vi "Swerve Wheel 6181.vi"(2 "Wheel":T1(ring), 4 "Inputs":dbl[](array[numeric])) -> (0 "Speed":dbl)   [LabVIEW 2019]
doc: "This vi is used to calculate and control the position of the swerve wheels and the commanded output to the drive motors."
uses:
  <vilib>/Rock Robotics/WPI/Utilities/WPI_GetSetVariantRefNum.vi
  <vilib>/addons/control/pid/pid.llb/PID (DBL).vi
  <vilib>/addons/control/pid/NI_PID_pid.lvlib
panel:
  in  "BR":dbl=245.0 format="%#_13g"
  in  "BL":dbl=95.0 format="%#_13g"
  in  "FR":dbl=267.0 format="%#_13g"
  in  "FL":dbl=75.0 format="%#_13g"
  # "Steering Motor Encoder Offsets"
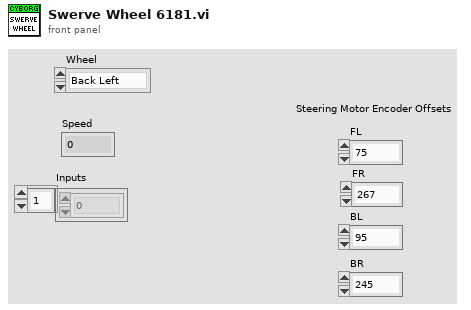
[diagram p1: front panel]
types:
  T1 = enum16{"Back Left", "Back Right", "Front Left", "Front Right"}
  T2 = enum16{"Z", "Y", "X", "Width/2", "Length/2", "Max"}
  T3 = cluster{"proportional gain (Kc)":dbl, "integral time (Ti, min)":dbl, "derivative time (Td, min)":dbl}
  T4 = typedef "WPI_AnalogChannelDevRef.ctl" = cluster{"DevStatus":errorcluster, "Analog Channel":T5}
  T5 = typedef "FPGA_AIChannel.ctl" = enum8{"AI 0", "AI 1", "AI 2", "AI 3", "AI MXP 0", "AI MXP 1", "AI MXP 2", "AI MXP 3", "Invalid"}
  T6 = typedef "WPI_MotorControlDeviceRef.ctl" = cluster{"DeviceStatus":errorcluster, "Type":T7, "PWM":cluster{"PWM Channel":T8, "DeadBand":T9}, "CAN":cluster{"Device Number":u8, "SetOutput VI Ref":variant, "GetOutput VI Ref":variant, "Enable VI Ref":variant, "Disable VI Ref":variant, "Data":variant}, "Invert":bool, "DIO PWM":cluster{"PWM \"Enable\" Channel":T8, "DIOChannel":T10, "PWM Rate":dbl}}
  T7 = typedef "WPI_MotorControlType.ctl" = enum16{"PWM", "CAN", "DIO PWM"}
  T8 = typedef "FPGA_DIOPWMChannel.ctl" = enum8{"PWM 0", "PWM 1", "PWM 2", "PWM 3", "PWM 4", "PWM 5", "PWM 6", "PWM 7", "PWM 8", "PWM 9", "PWM MXP 0", "PWM MXP 1", "PWM MXP 2", "PWM MXP 3", "PWM MXP 4", "PWM MXP 5", "PWM MXP 6", "PWM MXP 7", "PWM MXP 8", "PWM MXP 9", "Invalid"}
  T9 = typedef "WPI_PWMDeadband.ctl" = cluster{"Name":string, "maxPositivePwm":i32, "minPositivePwm":i32, "centerPwm":i32, "maxNegativePwm":i32, "minNegativePwm":i32, "angularRange":u16}
  T10 = typedef "FPGA_DIOChannel.ctl" = enum8{"DIO 0", "DIO 1", "DIO 2", "DIO 3", "DIO 4", "DIO 5", "DIO 6", "DIO 7", "DIO 8", "DIO 9", "DIO MXP 0", "DIO MXP 1", "DIO MXP 2", "DIO MXP 3", "DIO MXP 4", "DIO MXP 5", "DIO MXP 6", "DIO MXP 7", "DIO MXP 8", "DIO MXP 9", "DIO MXP 10", "DIO MXP 11", "DIO MXP 12", "DIO MXP 13", "DIO MXP 14", "DIO MXP 15", "SPI Port CS1", "SPI Port CS2", "SPI Port CS3", "SPI Port MISO", "SPI Port MOSI", "Invalid"}
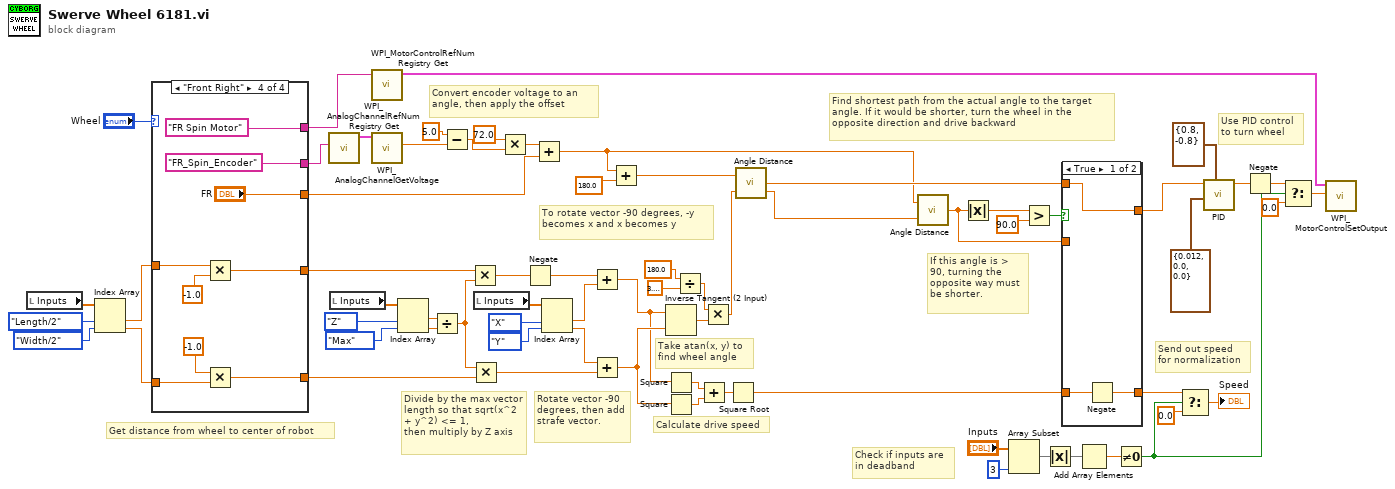
[diagram p0: block diagram]
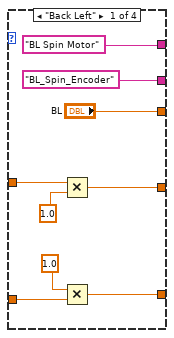
[diagram p3: hidden frame]
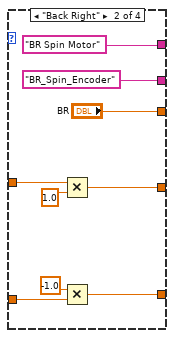
[diagram p4: hidden frame]
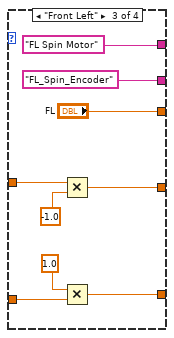
[diagram p5: hidden frame]
diagram:
  # "To rotate vector -90 degrees, -y becomes x and x becomes y"
  # "Divide by the max vector length so that sqrt(x^2 + y^2) <= 1,\nthen multiply by Z axis"
  # "Send out speed\nfor normalization"
  # "Check if inputs are\nin deadband"
  # "Convert encoder voltage to an angle, then apply the offset"
  # "If this angle is > 90, turning the opposite way must be shorter."
  # "Use PID control\nto turn wheel"
  # "Find shortest path from the actual angle to the target angle. If it would be shorter, turn the wheel in the opposite direction and drive backward"
  # "Take atan(x, y) to find wheel angle"
  # "Calculate drive speed"
  # "Rotate vector -90 degrees, then add strafe vector."
  # "Get distance from wheel to center of robot"
  n1 = local read "Inputs"() -> (w20:dbl[])
  n2 = Index Array(array=w20, index #1=T2."Length/2", index #2=T2."Width/2") -> (element #1=w19:dbl, element #2=w18:dbl)
  n3 = case shown="\"Front Right\"" "Wheel" {
    tunnel: ["BL_Spin_Encoder" "BR_Spin_Encoder" "FL_Spin_Encoder" "FR_Spin_Encoder"] -> w4
    tunnel: ["BL Spin Motor" "BR Spin Motor" "FL Spin Motor" "FR Spin Motor"] -> w3
    tunnel: ["BL" "BR" "FL" "FR"] -> w47
    tunnel: w19 -> [w73 w82 w91 w100]
    tunnel: w18 -> [w71 w80 w89 w98]
    tunnel: [w70 w79 w88 w97] -> w34
    tunnel: [w69 w78 w87 w96] -> w33
    frame "Back Left" {
      n4 = Multiply(x=w73, y=1.0) -> (x*y=w70:dbl)
      n5 = Multiply(x=1.0 ("y"), y=w71) -> (x*y=w69:dbl)
    }
    frame "Back Right" {
      n6 = Multiply(x=w82, y=1.0) -> (x*y=w79:dbl)
      n7 = Multiply(x=-1.0 ("y"), y=w80) -> (x*y=w78:dbl)
    }
    frame "Front Left" {
      n8 = Multiply(x=w91, y=-1.0) -> (x*y=w88:dbl)
      n9 = Multiply(x=1.0 ("y"), y=w89) -> (x*y=w87:dbl)
    }
    frame "Front Right" {
      n10 = Multiply(x=w100, y=-1.0) -> (x*y=w97:dbl)
      n11 = Multiply(x=-1.0 ("y"), y=w98) -> (x*y=w96:dbl)
    }
  }
  n12 = call <vilib>:"WPI_AnalogChannelRefNum Registry Get.vi"("refnum name"=w4) -> ("AIDeviceRef"=w50:T4)  [unwired: 9 in, 1 out]
  n13 = local read "Inputs"() -> (w32:dbl[])
  n14 = call <vilib>:"WPI_MotorControlRefNum Registry Get.vi"("refnum name"=w3) -> ("MotorControlDevRef"=w65:T6)  [unwired: 9 in, 1 out]
  n15 = call <vilib>:"WPI_AnalogChannelGetVoltage.vi"("AIDeviceRef"=w50) -> ("Voltage"=w13:dbl)  [unwired: 8 in, 2 out]
  n16 = Index Array(array=w32, index #1=T2."Z", index #2=T2."Max") -> (element #1=w30:dbl, element #2=w31:dbl)
  n17 = Divide(x=w30, y=w31) -> (x/y=w29:dbl)
  n18 = Subtract(x=5.0, y=w13) -> (x-y=w5:dbl)
  n19 = Multiply(x=w34, y=w29) -> (x*y=w16:dbl)
  n20 = Multiply(x=w29, y=w33) -> (x*y=w26:dbl)
  n21 = local read "Inputs"() -> (w28:dbl[])
  n22 = Multiply(x=72.0 ("y"), y=w5) -> (x*y=w48:dbl)
  n23 = Negate(x=w16) -> (-x=w15:dbl)
  n24 = Add(x=w48, y=w47) -> (x+y=w1:dbl)
  n25 = Index Array(array=w28, index #1=T2."X", index #2=T2."Y") -> (element #1=w24:dbl, element #2=w25:dbl)
  n26 = Add(x=w15, y=w24) -> (x+y=w22:dbl)
  n27 = Add(x=w25, y=w26) -> (x+y=w23:dbl)
  n28 = Add(x=w1, y=180.0 ("f")) -> (x+y=w43:dbl)
  n29 = Inverse Tangent (2 Input)(1:w23, 2:w22) -> (0:w63:dbl)
  n30 = Square(x=w22) -> (x^2=w27:dbl)
  n31 = Square(x=w23) -> (x^2=w62:dbl)
  n32 = Divide(x=180.0 ("y"), y=3.141592653589793) -> (x/y=w60:dbl)
  n33 = Add(x=w27, y=w62) -> (x+y=w61:dbl)
  n34 = Multiply(x=w60, y=w63) -> (x*y=w17:dbl)
  n35 = Square Root(x=w61) -> (sqrt(x)=w54:dbl)
  n36 = call "Angle Distance.vi"("target angle"=w17, "current angle"=w43) -> ("distance"=w6:dbl)
  n37 = call "Angle Distance.vi"("target angle"=w17, "current angle"=w1) -> ("distance"=w55:dbl)
  n38 = Absolute Value(x=w55) -> (abs(x)=w56:dbl)
  n39 = Array Subset(array="Inputs", length=3) -> (w42:dbl[])  [unwired: 1 in]
  n40 = Greater?(x=w56, y=90.0) -> (0:w38:bool)
  n41 = Absolute Value(x=w42) -> (abs(x)=w35:dbl[])
  n42 = case shown="True" w38 {
    tunnel: w6 -> [w104 _]
    tunnel: w55 -> [_ w108]
    tunnel: [w105 w107] -> w41
    tunnel: w54 -> [w106 w107]
    tunnel: [w104 w108] -> w51
    frame True {
      n43 = Negate(x=w106) -> (-x=w105:dbl)
    }
    frame False {
    }
  }
  n44 = Add Array Elements(numeric array=w35) -> (sum=w64:dbl)
  n45 = Not Equal To 0?(x=w64) -> (x != 0?=w37:bool)
  n46 = Select(t=w41, s=w37, f=0.0) -> (s? t:f=→"Speed":dbl)
  n47 = call-poly <vilib>:"PID.vi"("output range"=cluster{"output high":dbl, "output low":dbl} {"output high"=0.8, "output low"=-0.8}, "PID gains"=T3 {"proportional gain (Kc)"=0.012, "integral time (Ti, min)"=0.0, "derivative time (Td, min)"=0.0}, "setpoint"=w51) -> ("output"=w45:dbl)  [unwired: 7 in, 1 out]
  n48 = Negate(x=w45) -> (-x=w36:dbl)
  n49 = Select(t=w36, s=w37, f=0.0) -> (s? t:f=w46:dbl)
  n50 = call <vilib>:"WPI_MotorControlSetOutput.vi"("Output"=w46, "MotorControlDevRef"=w65) -> ()  [unwired: 7 in, 3 out]
